vi "WPI_RobotDriveArcadeDrive_Standard(NoSaturation)2.vi"(8 "error in (no error)":errorcluster, 9 "Y axis value":dbl, 10 "X axis value":dbl, 11 "RobotDriveDevRef":T1={"DevStatus"={"status"=FALSE, "code"=0, "source"=""}, "Motors[]"=[], "Square Inputs"=FALSE, "Max Output"=1.0, "Isochronous"=FALSE}) -> (0 "error out":errorcluster, 3 "RobotDriveDevRef":T1={"DevStatus"={"status"=FALSE, "code"=0, "source"=""}, "Motors[]"=[], "Square Inputs"=FALSE, "Max Output"=1.0, "Isochronous"=FALSE})   [LabVIEW 2012]
doc: "Uses a standard algorithm to configure the motors for arcade driving. This algorithm does not saturate over half of the range.\n\nThis software is licensed. Open the labview\\readme\\WPI Robotics Library Open Source License.txt file for more information."
uses:
  <vilib>/Rock Robotics/WPI/RobotDrive/WPI_RobotDriveDevRef.ctl
  <vilib>/Rock Robotics/WPI/MotorControl/WPI_MotorControlDeviceRef.ctl
  <vilib>/Rock Robotics/SystemInterfaces/Typedef/FPGA_TypedefDigitalModule.ctl
  <vilib>/Rock Robotics/SystemInterfaces/DIO/FPGA_DIOPWMChannel.ctl
  <vilib>/Rock Robotics/WPI/PWM/WPI_PWMDeadband.ctl
  <vilib>/Rock Robotics/WPI/CAN/Jaguar/SubVIs/WPI_CANJaguar_ControlMode.ctl
  <vilib>/Rock Robotics/WPI/PWM/WPI_PWMTransform_ConPane.ctl
  <vilib>/Rock Robotics/SystemInterfaces/NetworkCommunication/NetComm_UsageReport_ResourceType.ctl
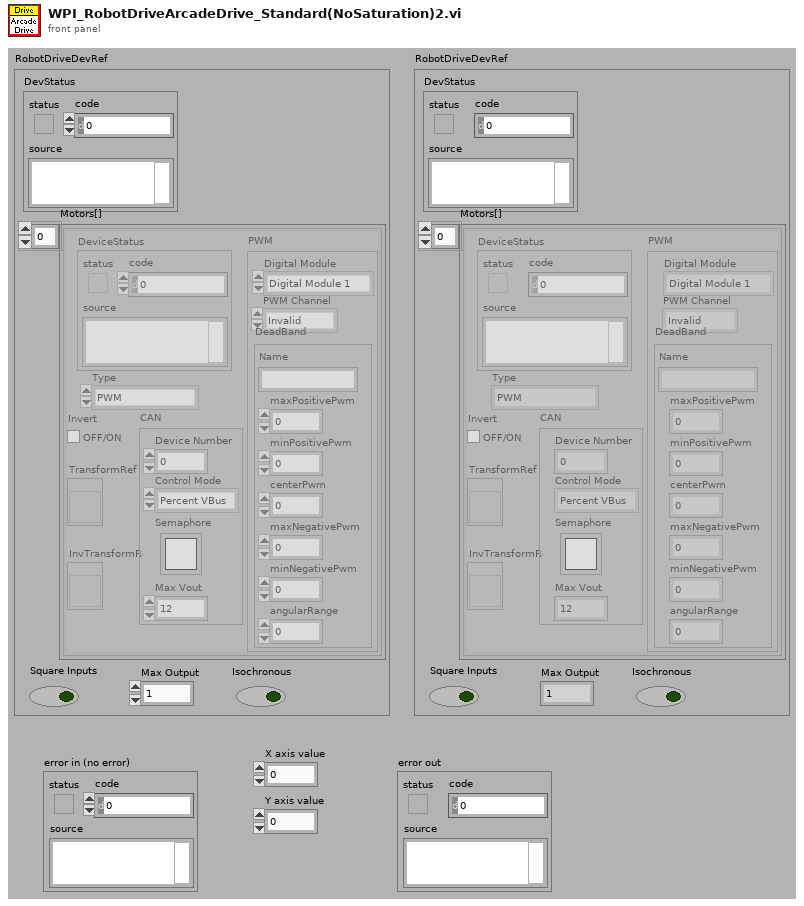
[diagram p1: front panel]
types:
  T1 = typedef "WPI_RobotDriveDevRef.ctl" = cluster{"DevStatus":errorcluster, "Motors[]":T2[], "Square Inputs":bool, "Max Output":dbl, "Isochronous":bool}
  T2 = typedef "WPI_MotorControlDeviceRef.ctl" = cluster{"DeviceStatus":errorcluster, "Type":enum16{"PWM", "CAN"}, "PWM":cluster{"Digital Module":T3, "PWM Channel":T4, "DeadBand":T5}, "CAN":cluster{"Device Number":u8, "Control Mode":T6, "Semaphore":T7, "Max Vout":dbl}, "Invert":bool, "TransformRef":T8, "InvTransformRef":T8}
  T3 = typedef "FPGA_TypedefDigitalModule.ctl" = enum16{"Digital Module 1", "Digital Module 2"}
  T4 = typedef "FPGA_DIOPWMChannel.ctl" = enum8{"PWM 1", "PWM 2", "PWM 3", "PWM 4", "PWM 5", "PWM 6", "PWM 7", "PWM 8", "PWM 9", "PWM 10", "Invalid"}
  T5 = typedef "WPI_PWMDeadband.ctl" = cluster{"Name":string, "maxPositivePwm":i32, "minPositivePwm":i32, "centerPwm":i32, "maxNegativePwm":i32, "minNegativePwm":i32, "angularRange":u16}
  T6 = typedef "WPI_CANJaguar_ControlMode.ctl" = enum8{"Percent VBus", "Current", "Speed", "Position", "Voltage"}
  T7 = typedef "Semaphore RefNum" = refnum<k1>
  T8 = typedef "WPI_PWMTransform_ConPane.ctl" = refnum<vi>
  T9 = typedef "NetComm_UsageReport_ResourceType.ctl" = enum8{"Controller", "Module", "Language", "CANPlugin", "Accelerometer", "ADXL345", "AnalogChannel", "AnalogTrigger", "AnalogTriggerOutput", "CANJaguar", "Compressor", "Counter", "Dashboard", "DigitalInput", "DigitalOutput", "DriverStationCIO", "DriverStationEIO", "DriverStationLCD", "Encoder", "GearTooth", "Gyro", "I2C", "Framework", "Jaguar", "Joystick", "Kinect", "KinectStick", "PIDController", "Preferences", "PWM", "Relay", "RobotDrive", "SerialPort", "Servo", "Solenoid", "SPI", "Task", "Ultrasonic", "Victor", "Button", "Command", "AxisCamera", "PCVideoServer", "SmartDashboard", "Talon", "HiTechnicColorSensor", "HiTechnicAccel", "HiTechnicCompass", "SRF08"}
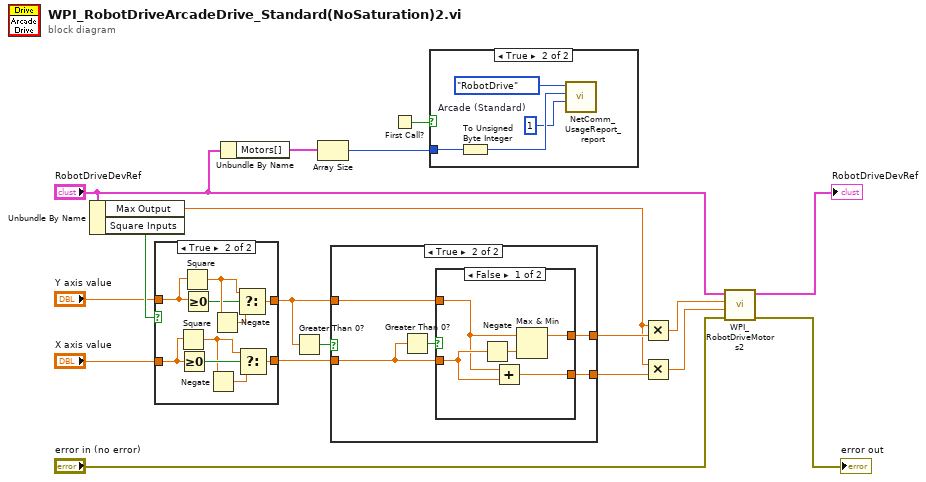
[diagram p0: block diagram]
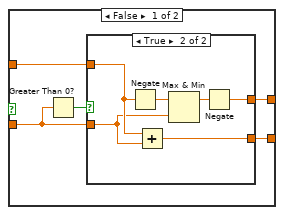
[diagram p3: hidden frame]
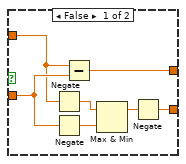
[diagram p4: hidden frame]
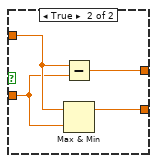
[diagram p5: hidden frame]
diagram:
  n1 = Unbundle By Name("RobotDriveDevRef") -> ("Max Output"=w7:dbl, "Square Inputs"=w17:bool)
  n2 = case shown="True" w17 {
    tunnel: [w19 w30] -> w14
    tunnel: [w20 w29] -> w15
    tunnel: "X axis value" -> [w19 w28]
    tunnel: "Y axis value" -> [w20 w27]
    frame False {
    }
    frame True {
      n3 = Square(x=w28) -> (x^2=w25:dbl)
      n4 = Greater Or Equal To 0?(x=w28) -> (x >= 0?=w26:bool)
      n5 = Square(x=w27) -> (x^2=w22:dbl)
      n6 = Greater Or Equal To 0?(x=w27) -> (x >= 0?=w21:bool)
      n7 = Negate(x=w25) -> (-x=w24:dbl)
      n8 = Negate(x=w22) -> (-x=w23:dbl)
      n9 = Select(t=w22, s=w21, f=w23) -> (s? t:f=w29:dbl)
      n10 = Select(t=w25, s=w26, f=w24) -> (s? t:f=w30:dbl)
    }
  }
  n11 = Unbundle By Name("RobotDriveDevRef") -> ("Motors[]"=w2:T2[])
  n12 = Greater Than 0?(x=w15) -> (x > 0?=w16:bool)
  n13 = Array Size(array=w2) -> (size(s)=w1:i32)
  n14 = case shown="True" w16 {
    tunnel: w14 -> [w34 w52]
    tunnel: w15 -> [w33 w51]
    tunnel: [w32 w50] -> w13
    tunnel: [w31 w49] -> w9
    frame False {
      n15 = Greater Than 0?(x=w34) -> (x > 0?=w35:bool)
      n16 = case shown="True" w35 {
        tunnel: w34 -> [w42 w44]
        tunnel: w33 -> [w40 w45]
        tunnel: [w36 w46] -> w32
        tunnel: [w37 w43] -> w31
        frame False {
          n17 = Negate(x=w40) -> (-x=w41:dbl)
          n18 = Negate(x=w42) -> (-x=w39:dbl)
          n19 = Subtract(x=w40, y=w42) -> (x-y=w36:dbl)
          n20 = Max & Min(x=w41, y=w39) -> (max(x,y)=w38:dbl)  [unwired: 1 out]
          n21 = Negate(x=w38) -> (-x=w37:dbl)
        }
        frame True {
          n22 = Negate(x=w45) -> (-x=w48:dbl)
          n23 = Add(x=w45, y=w44) -> (x+y=w43:dbl)
          n24 = Max & Min(x=w48, y=w44) -> (max(x,y)=w47:dbl)  [unwired: 1 out]
          n25 = Negate(x=w47) -> (-x=w46:dbl)
        }
      }
    }
    frame True {
      n26 = Greater Than 0?(x=w52) -> (x > 0?=w53:bool)
      n27 = case shown="False" w53 {
        tunnel: w52 -> [w58 w60]
        tunnel: w51 -> [w55 w61]
        tunnel: [w56 w59] -> w50
        tunnel: [w54 w62] -> w49
        frame False {
          n28 = Negate(x=w58) -> (-x=w57:dbl)
          n29 = Add(x=w55, y=w58) -> (x+y=w54:dbl)
          n30 = Max & Min(x=w55, y=w57) -> (max(x,y)=w56:dbl)  [unwired: 1 out]
        }
        frame True {
          n31 = Subtract(x=w61, y=w60) -> (x-y=w59:dbl)
          n32 = Max & Min(x=w61, y=w60) -> (max(x,y)=w62:dbl)  [unwired: 1 out]
        }
      }
    }
  }
  n33 = First Call?() -> (First Call?: T/F=w4:bool)
  n34 = case shown="True" w4 {
    tunnel: w1 -> [_ w65]
    frame False {
    }
    frame True {
      w63 = u8 1  # Arcade (Standard)
      n35 = To Unsigned Byte Integer(number=w65) -> (unsigned 8bit integer=w64:u8)
      n36 = call <vilib>:"NetComm_UsageReport_report.vi"("Context"=w63, "Instance Number"=w64, "Resource Type"=NetComm_UsageReport_ResourceType."RobotDrive") -> ()  [unwired: 9 in]
    }
  }
  n37 = Multiply(x=w7, y=w13) -> (x*y=w10:dbl)
  n38 = Multiply(x=w7, y=w9) -> (x*y=w8:dbl)
  n39 = call "WPI_RobotDriveMotors2.vi"("error in (no error)"="error in (no error)", "RightSpeed"=w8, "LeftSpeed"=w10, "RobotDriveDevRef"="RobotDriveDevRef") -> ("error out"=→"error out":errorcluster, "RobotDriveDevRef"=→"RobotDriveDevRef":T1)  [unwired: 6 in]
